vi "Sonicator Settings Dialog.vi"(8 "error in (no error)":errorcluster, 10 "Message Queues":T1, 11 "Sonicator Module State Cluster":T5={"State"=enum."Idle", "Start Time"=timestamp(0 s since 1904-01-01), "Current Time"=timestamp(0 s since 1904-01-01), "Sonicator Module Config"={"GUID"="", "Drop Coords"={"Horizontal"=0, "Vertical"=0}, "Process Name"="", "Queue Name"="", "Settings"={"Cycle Period"=500.0, "Sonicator Type"="Sonic Systems P100", "SS P100 Settings"={"VISA resource name"="", "Simulated?"=FALSE}, "Setpoint (µm)"=0.0, "Cutoff (µm)"=0.0}, "Load Count"=0}, "Output Error"=FALSE, "Log Started"=FALSE, "First Iteration"=FALSE, "Data"={"Sonicator Amp Value"=0.0, "Sonicator Power Value"=0.0}, "Sonicator On?"=enum."Off"}) -> (0 "error out":errorcluster, 1 "Cancelled?":bool=TRUE, 2 "UI Refresh Needed?":bool, 3 "Sonicator Module State Cluster":T5={"State"=enum."Idle", "Start Time"=timestamp(0 s since 1904-01-01), "Current Time"=timestamp(0 s since 1904-01-01), "Sonicator Module Config"={"GUID"="", "Drop Coords"={"Horizontal"=0, "Vertical"=0}, "Process Name"="", "Queue Name"="", "Settings"={"Cycle Period"=500.0, "Sonicator Type"="Sonic Systems P100", "SS P100 Settings"={"VISA resource name"="", "Simulated?"=FALSE}, "Setpoint (µm)"=0.0, "Cutoff (µm)"=0.0}, "Load Count"=0}, "Output Error"=FALSE, "Log Started"=FALSE, "First Iteration"=FALSE, "Data"={"Sonicator Amp Value"=0.0, "Sonicator Power Value"=0.0}, "Sonicator On?"=enum."Off"})   [LabVIEW 2018, in "Sonicator Module.lvlib"]
doc: "Dialog for selecting user specified settings."
uses:
  Sonicator Module.lvlib
  Feed Module/Controls/Sonicator Module State Cluster.ctl
  Pump Module Folder/Measure Instrument/State Enum.ctl
  Feed Module/Controls/Sonicator Module Config Cluster.ctl
  <vilib>/Utility/miscctls.llb/LVPoint32TypeDef.ctl
  Feed Module/Controls/Sonicator Module Settings Cluster.ctl
  Sonic Systems P100/Sonic Systems P100 Settings.ctl
  Feed Module/Controls/Sonicator Module Settings Cluster and Start Stop.ctl
  Sonicator Message Queues.ctl
  support/Message Queue/Message Cluster.ctl
  support/Message Queue/Enqueue Message (Single).vi
  <vilib>/Utility/xml.llb/Write to XML File(string).vi
  Settings/Settings.lvlib
  Measure Instrument/Sonicator Module Engine.lvlib
  support/Support Library.lvlib
  support/Message Queue/Message Queue.lvlib
  Sonic Systems P100/Sonic Systems P100.lvlib
  Pump Module Folder/Measure Instrument/Pump Module Engine.lvlib
panel:
  in  "Configuration + Buttons":T2={"Configuration"={"Cycle Period"=500.0, "Sonicator Type"="", "SS P100 Settings"={"VISA resource name"="", "Simulated?"=FALSE}, "Setpoint (µm)"=0.0, "Cutoff (µm)"=0.0}, "Stop"=FALSE, "Start"=FALSE}
  in  "Module Name":string
  in  "Cancel Button":bool
  in  "OK Button":bool
  # "Non visible portion of dialog (needed for connector pane)."
  # "Sonicator Settings"
  # "Sonicator Settings"
  # "Sonicator Settings"
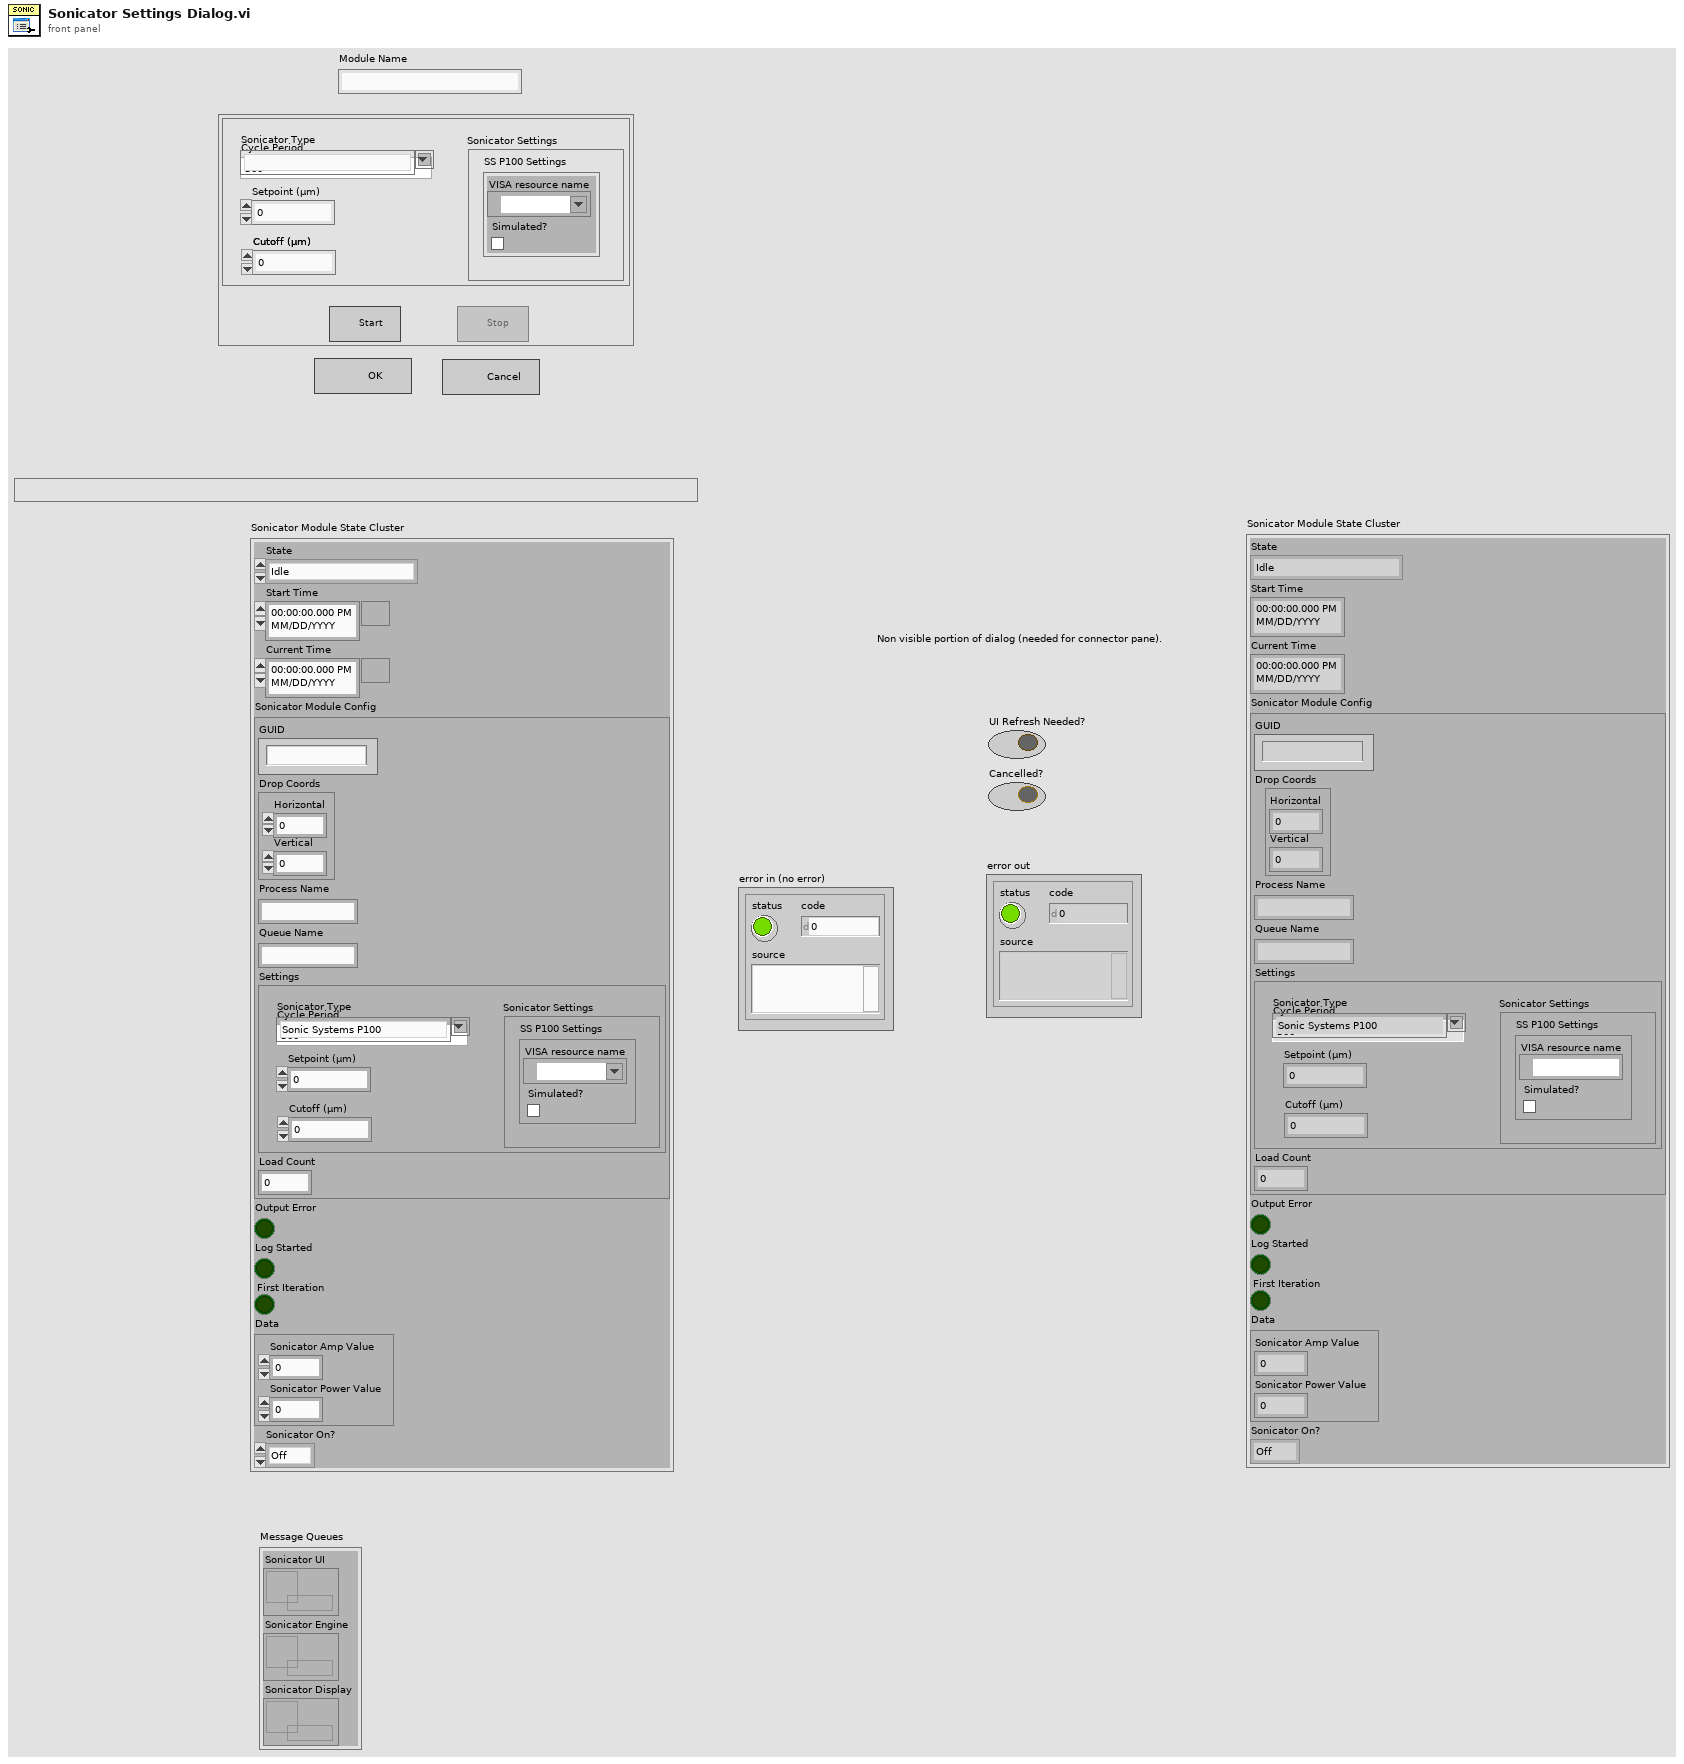
[diagram p1: front panel]
types:
  T1 = typedef "Sonicator Module.lvlib/Sonicator Message Queues.ctl" = cluster{"Sonicator UI":refnum<queue>, "Sonicator Engine":refnum<queue>, "Sonicator Display":refnum<queue>}
  T2 = typedef "Sonicator Module.lvlib/Sonicator Module Settings Cluster and Start Stop.ctl" = cluster{"Configuration":T3, "Stop":bool, "Start":bool}
  T3 = typedef "Sonicator Module.lvlib/Sonicator Module Settings Cluster.ctl" = cluster{"Cycle Period":dbl, "Sonicator Type":string, "SS P100 Settings":T4, "Setpoint (µm)":dbl, "Cutoff (µm)":dbl}
  T4 = typedef "Sonic Systems P100.lvlib/Sonic Systems P100 Settings.ctl" = cluster{"VISA resource name":refnum<visa-resource-name>, "Simulated?":bool}
  T5 = typedef "Sonicator Module.lvlib/Sonicator Module State Cluster.ctl" = cluster{"State":T6, "Start Time":timestamp, "Current Time":timestamp, "Sonicator Module Config":T7, "Output Error":bool, "Log Started":bool, "First Iteration":bool, "Data":cluster{"Sonicator Amp Value":dbl, "Sonicator Power Value":dbl}, "Sonicator On?":enum16{"Off", "On", "Not Initialized", "Over Cutoff"}}
  T6 = typedef "Pump Module.lvlib/Pump Module Engine.lvlib/State Enum.ctl" = enum16{"Measuring", "Idle", "Paused"}
  T7 = typedef "Sonicator Module.lvlib/Sonicator Module Config Cluster.ctl" = cluster{"GUID":string, "Drop Coords":T8, "Process Name":string, "Queue Name":string, "Settings":T3, "Load Count":i32}
  T8 = typedef "LVPoint32TypeDef.ctl" = cluster{"Horizontal":i32, "Vertical":i32}
  T9 = enum8{"Enabled", "Disabled", "Disabled and Grayed Out"}
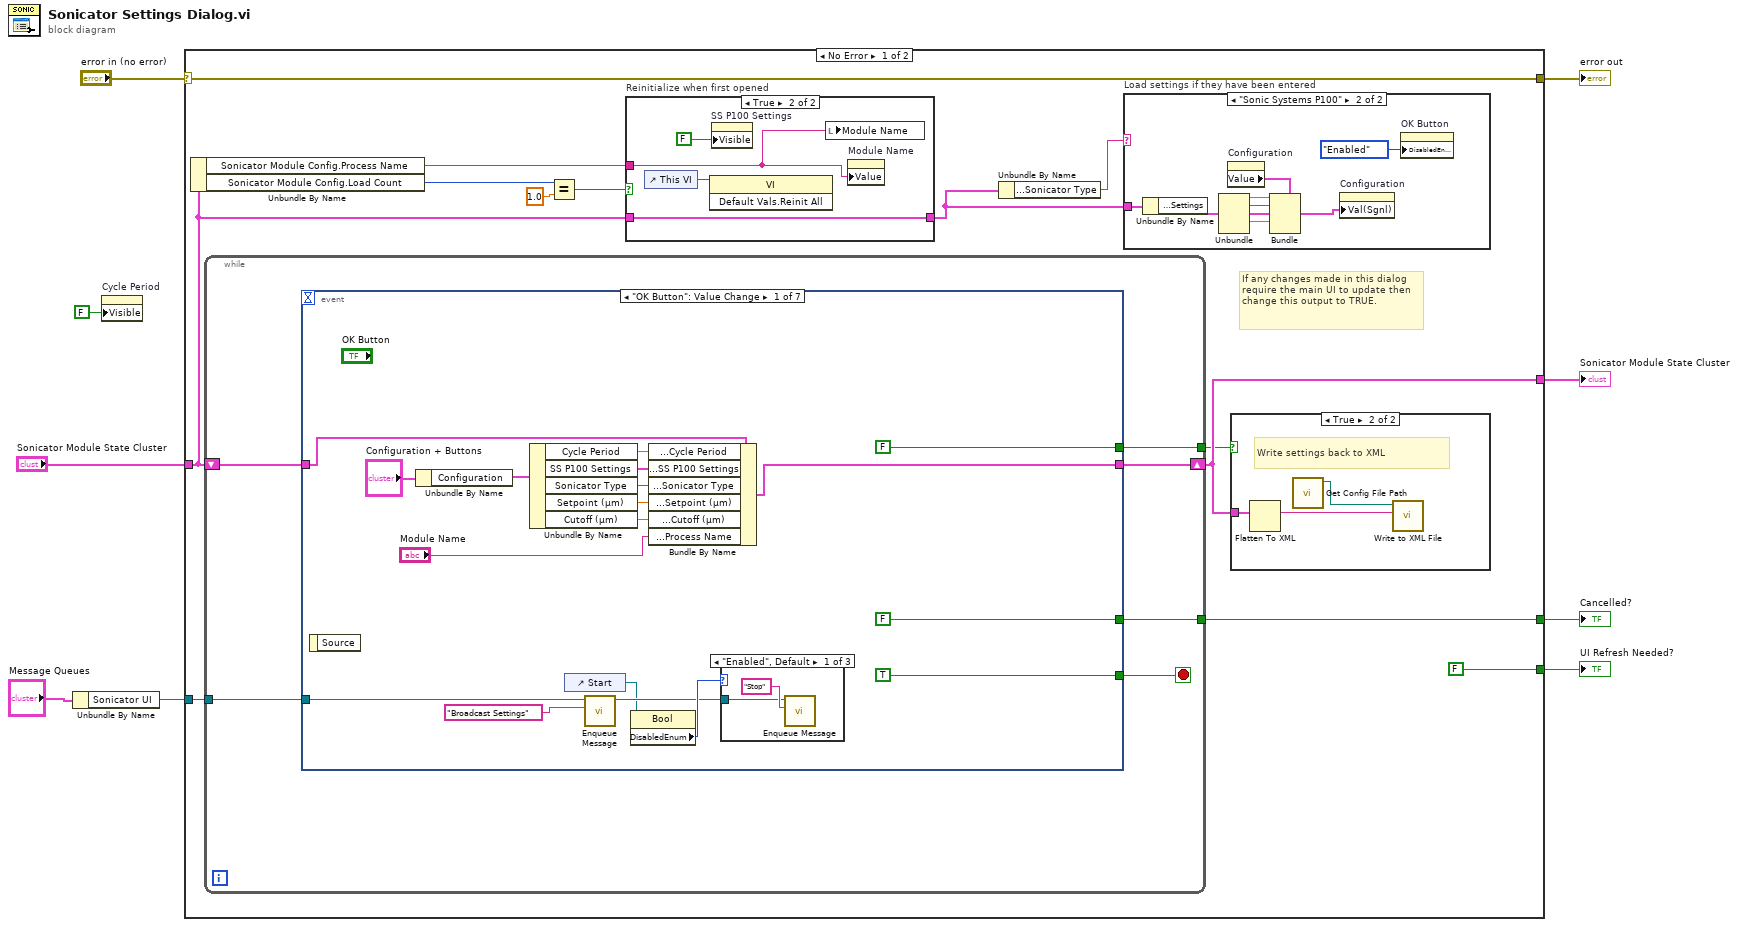
[diagram p0: block diagram]
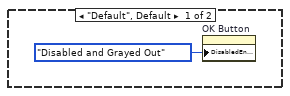
[diagram p2: hidden frame]
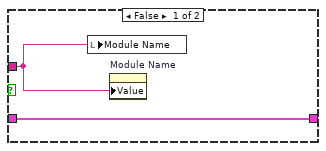
[diagram p3: hidden frame]
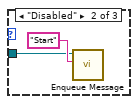
[diagram p4: hidden frame]
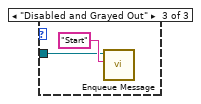
[diagram p5: hidden frame]
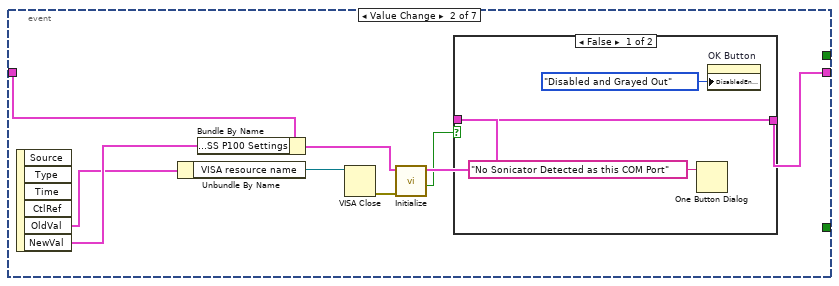
[diagram p6: hidden frame]
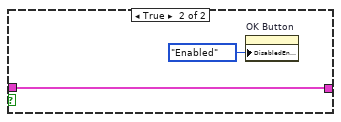
[diagram p7: hidden frame]
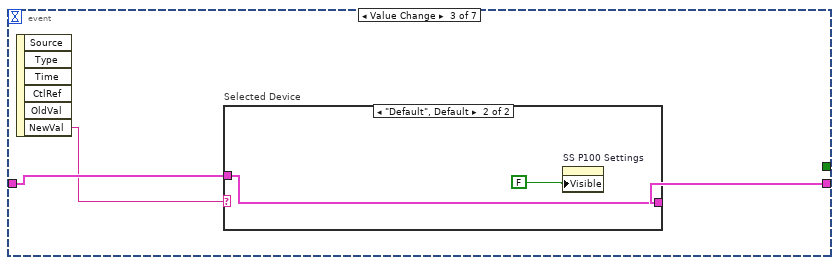
[diagram p8: hidden frame]
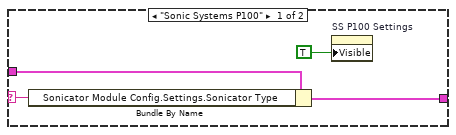
[diagram p9: hidden frame]
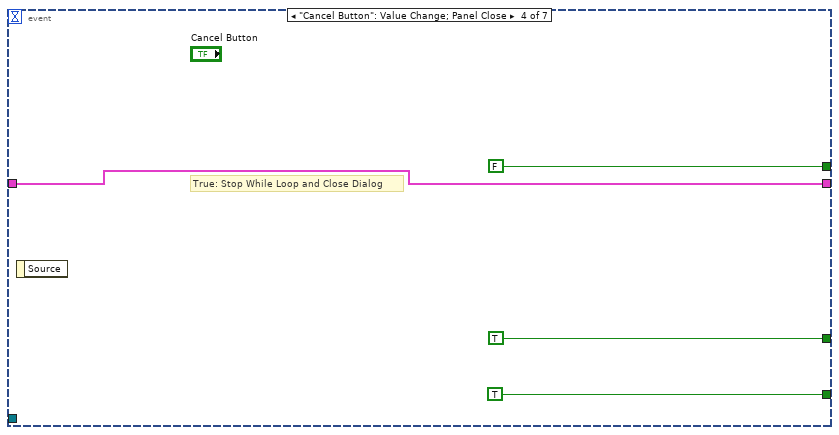
[diagram p10: hidden frame]
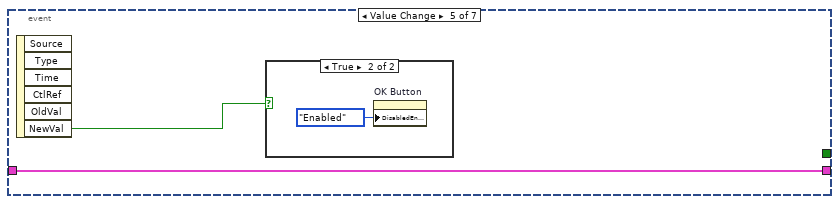
[diagram p11: hidden frame]
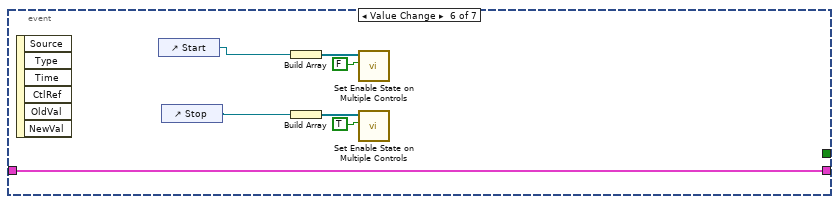
[diagram p13: hidden frame]
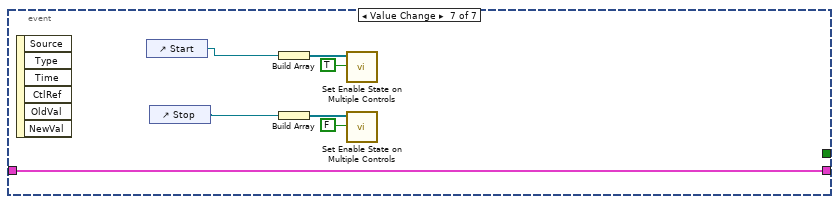
[diagram p14: hidden frame]
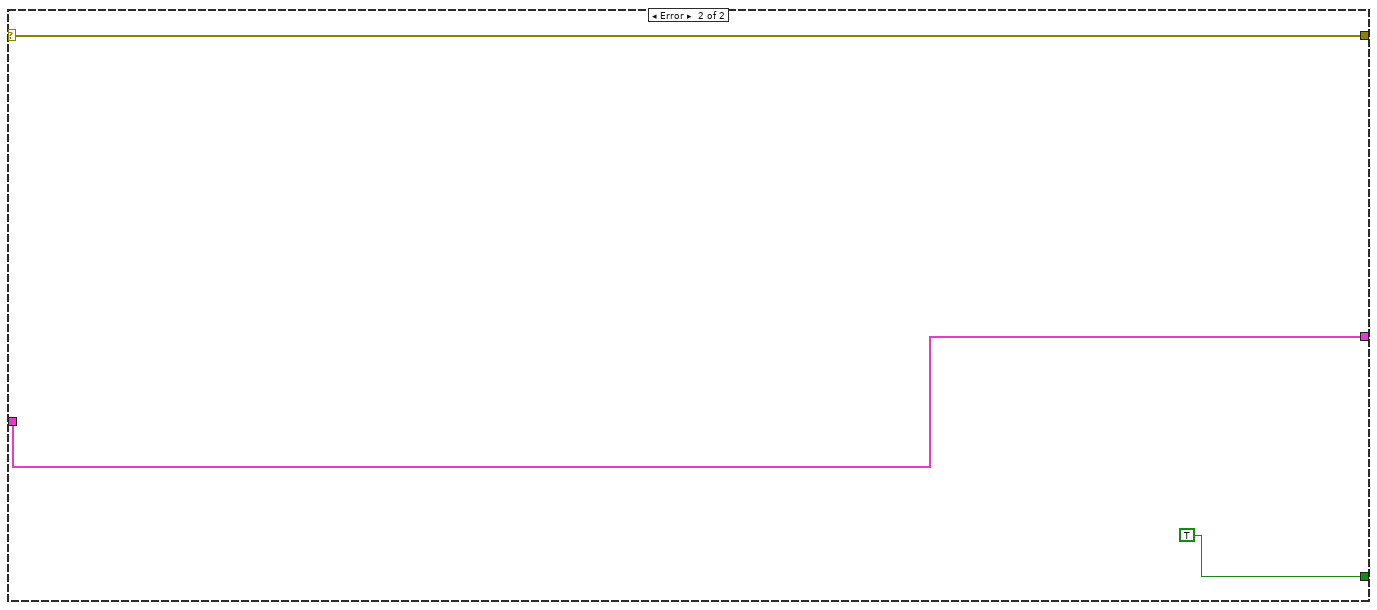
[diagram p16: hidden frame]
diagram:
  n1 = Unbundle By Name("Message Queues") -> ("Sonicator UI"=w1:refnum<queue>)
  n2 = property on="Cycle Period" class="DigNum (strict)"("Visible"=FALSE) -> ()  [unwired: 2 in, 2 out]
  n3 = case shown="No Error" "error in (no error)" {
    selector: "error in (no error)" -> [w22 w118]
    tunnel: [w22 w118] -> w9
    tunnel: "Sonicator Module State Cluster" -> [w12 w117]
    tunnel: [w20 w117] -> w4
    tunnel: [FALSE ("UI Refresh Needed?") _] -> w8
    tunnel: [w16 TRUE ("UI Refresh Needed?")] -> w7
    tunnel: w1 -> [w10 _]
    frame No Error {
      # "If any changes made in this dialog require the main UI to update then change this output to TRUE."
      n4 = Unbundle By Name(w12) -> ("Sonicator Module Config.Process Name"=w11:string, "Sonicator Module Config.Load Count"=w19:i32)
      n5 = while {
        tunnel: [w44] -> w17
        tunnel: [w41] -> w16
        shift-right: [w43] -> w20
        shift-left: w12 -> [w40]
        tunnel: w10 -> [w39]
        stop <- w42 stop-if-true
        n6 = event shown="[0] \"OK Button\": Value Change" {
          selector: _ -> [_ _ _ _ _ _ _]
          dyn-events: _ -> [_ _ _ _ _ _ _]
          timeout: _ -> [_ _ _ _ _ _ _]
          tunnel: [w60 w77 w83 w95 w97 w105 w112] -> w43
          tunnel: w40 -> [w57 w75 w85 w95 w97 w105 w112]
          tunnel: [FALSE ("UI Refresh Needed?") _ _ FALSE ("UI Refresh Needed?") _ _ _] -> w44
          tunnel: [TRUE _ _ TRUE _ _ _] -> w42
          tunnel: [FALSE ("UI Refresh Needed?") _ _ TRUE ("UI Refresh Needed?") _ _ _] -> w41
          tunnel: w39 -> [w47 _ _ _ _ _ _]
          event "OK Button": Value Change {
            n7 = event-data() -> ()  [unwired: 1 in, 1 out]
            n8 = Unbundle By Name("Configuration + Buttons") -> ("Configuration"=w53:T3)
            n9 = Unbundle By Name(w53) -> ("Cycle Period"=w58:dbl, "SS P100 Settings"=w56:T4, "Sonicator Type"=w55:string, "Setpoint (µm)"=w52:dbl, "Cutoff (µm)"=w45:dbl)
            n10 = control-ref of="Start"() -> (w48:refnum<vi>)
            n11 = call-poly "Enqueue Message.vi"("Message"="Broadcast Settings", "Message Queue"=w47) -> ("dup Message Queue"=w49:refnum<queue>)  [unwired: 8 in, 1 out]
            n12 = property class="Bool"(reference=w48) -> ("DisabledEnum"=w51:T9)  [unwired: 1 in, 2 out]
            n13 = Bundle By Name(cluster=w57, "Sonicator Module Config.Settings.Cycle Period"=w58, "Sonicator Module Config.Settings.SS P100 Settings"=w56, "Sonicator Module Config.Settings.Sonicator Type"=w55, "Sonicator Module Config.Settings.Setpoint (µm)"=w52, "Sonicator Module Config.Settings.Cutoff (µm)"=w45, "Sonicator Module Config.Process Name"="Module Name") -> (w60:T5)
            n14 = case shown="\"Enabled\", Default" w51 {
              tunnel: w49 -> [w63 w65 w67]
              frame "Enabled", Default {
                n15 = call-poly "Enqueue Message.vi"("Message"="Stop", "Message Queue"=w63) -> ()  [unwired: 8 in, 2 out]
              }
              frame "Disabled" {
                n16 = call-poly "Enqueue Message.vi"("Message"="Start", "Message Queue"=w65) -> ()  [unwired: 8 in, 2 out]
              }
              frame "Disabled and Grayed Out" {
                n17 = call-poly "Enqueue Message.vi"("Message"="Start", "Message Queue"=w67) -> ()  [unwired: 8 in, 2 out]
              }
            }
          }
          event Value Change {
            n18 = event-data() -> ("OldVal"=w69:T4, "NewVal"=w71:T4)  [unwired: 1 in, 4 out]
            n19 = Unbundle By Name(w69) -> ("VISA resource name"=w70:refnum<visa-resource-name>)
            n20 = Bundle By Name(cluster=w75, "Sonicator Module Config.Settings.SS P100 Settings"=w71) -> (w74:T5)
            n21 = VISA Close(VISA resource name=w70) -> (error out=w76:errorcluster)  [unwired: 1 in]
            n22 = call "Initialize.vi"("error in (no error)"=w76, "Sonicator Module State Cluster"=w74) -> ("Initialized"=w72:bool, "Sonicator Module State Cluster"=w73:T5)  [unwired: 7 in, 1 out]
            n23 = case shown="False" w72 {
              tunnel: [w79 w81] -> w77
              tunnel: w73 -> [w79 w81]
              frame False {
                n24 = One Button Dialog(message="No Sonicator Detected as this COM Port") -> ()  [unwired: 1 in, 1 out]
                n25 = property on="OK Button" class="Bool"("DisabledEnum"=T9."Disabled and Grayed Out" ("Disabled")) -> ()  [unwired: 2 in, 2 out]
              }
              frame True {
                n26 = property on="OK Button" class="Bool"("DisabledEnum"=T9."Enabled" ("Disabled")) -> ()  [unwired: 2 in, 2 out]
              }
            }
          }
          event Value Change {
            n27 = event-data() -> ("NewVal"=w84:string)  [unwired: 1 in, 5 out]
            n28 = case "Selected Device" shown="\"Default\", Default" w84 {
              selector: w84 -> [w87 _]
              tunnel: w85 -> [w89 w91]
              tunnel: [w88 w91] -> w83
              frame "Sonic Systems P100" {
                n29 = Bundle By Name(cluster=w89, "Sonicator Module Config.Settings.Sonicator Type"=w87) -> (w88:T5)
                n30 = property on="SS P100 Settings" class="Clust (strict)"("Visible"=TRUE) -> ()  [unwired: 2 in, 2 out]
              }
              frame "Default", Default {
                n31 = property on="SS P100 Settings" class="Clust (strict)"("Visible"=FALSE) -> ()  [unwired: 2 in, 2 out]
              }
            }
          }
          event "Cancel Button": Value Change; Panel Close {
            # "True: Stop While Loop and Close Dialog"
            n32 = event-data() -> ()  [unwired: 1 in, 1 out]
          }
          event Value Change {
            n33 = event-data() -> ("NewVal"=w96:bool)  [unwired: 1 in, 5 out]
            n34 = case shown="True" w96 {
              frame False {
              }
              frame True {
                n35 = property on="OK Button" class="Bool"("DisabledEnum"=T9."Enabled" ("Disabled")) -> ()  [unwired: 2 in, 2 out]
              }
            }
          }
          event Value Change {
            n36 = event-data() -> ()  [unwired: 1 in, 6 out]
            n37 = control-ref of="Start"() -> (w100:refnum<vi>)
            n38 = control-ref of="Stop"() -> (w99:refnum<vi>)
            n39 = Build Array(w100) -> (w102:refnum<vi>[])
            n40 = Build Array(w99) -> (w104:refnum<vi>[])
            n41 = call "Set Enable State on Multiple Controls.vi"("Enable?"=FALSE, "Controls"=w102) -> ()  [unwired: 10 in]
            n42 = call "Set Enable State on Multiple Controls.vi"("Enable?"=TRUE, "Controls"=w104) -> ()  [unwired: 10 in]
          }
          event Value Change {
            n43 = event-data() -> ()  [unwired: 1 in, 6 out]
            n44 = control-ref of="Start"() -> (w109:refnum<vi>)
            n45 = control-ref of="Stop"() -> (w108:refnum<vi>)
            n46 = Build Array(w109) -> (w110:refnum<vi>[])
            n47 = Build Array(w108) -> (w111:refnum<vi>[])
            n48 = call "Set Enable State on Multiple Controls.vi"("Enable?"=TRUE, "Controls"=w110) -> ()  [unwired: 10 in]
            n49 = call "Set Enable State on Multiple Controls.vi"("Enable?"=FALSE, "Controls"=w111) -> ()  [unwired: 10 in]
          }
        }
      }
      n50 = Equal?(x=w19, y=1.0) -> (x = y?=w15:bool)
      n51 = case "Reinitialize when first opened" shown="True" w15 {
        tunnel: w12 -> [w34 w37]
        tunnel: [w34 w37] -> w13
        tunnel: w11 -> [w33 w36]
        frame False {
          n52 = local write "Module Name"(w33) -> ()
          n53 = property on="Module Name" class="Str"("Value"=w33) -> ()  [unwired: 2 in, 2 out]
        }
        frame True {
          n54 = control-ref of="This VI"() -> (w38:refnum<vi>)
          n55 = invoke class="VI" method="Default Vals.Reinit All"(reference=w38) -> ()  [unwired: 2 in, 3 out]
          n56 = property on="SS P100 Settings" class="Clust (strict)"("Visible"=FALSE) -> ()  [unwired: 2 in, 2 out]
          n57 = local write "Module Name"(w36) -> ()
          n58 = property on="Module Name" class="Str"("Value"=w36) -> ()  [unwired: 2 in, 2 out]
        }
      }
      n59 = Unbundle By Name(w13) -> ("Sonicator Module Config.Settings.Sonicator Type"=w14:string)
      n60 = case "Load settings if they have been entered" shown="\"Sonic Systems P100\"" w14 {
        tunnel: w13 -> [_ w28]
        frame "Default", Default {
          n61 = property on="OK Button" class="Bool"("DisabledEnum"=T9."Disabled and Grayed Out" ("Disabled")) -> ()  [unwired: 2 in, 2 out]
        }
        frame "Sonic Systems P100" {
          n62 = Unbundle By Name(w28) -> ("Sonicator Module Config.Settings"=w30:T3)
          n63 = Unbundle(w30) -> ("Cycle Period"=w31:dbl, "Sonicator Type"=w32:string, "SS P100 Settings"=w29:T4, "Setpoint (µm)"=w26:dbl)  [unwired: 1 out]
          n64 = property on="Configuration" class="Clust (strict)"() -> ("Value"=w25:T3)  [unwired: 2 in, 2 out]
          n65 = Bundle(cluster=w25, "Cycle Period"=w31, "Sonicator Type"=w32, "SS P100 Settings"=w29, "Setpoint (µm)"=w26) -> (w24:T3)  [unwired: 1 in]
          n66 = property on="Configuration" class="Clust (strict)"("Val(Sgnl)"=w24) -> ()  [unwired: 2 in, 2 out]
          n67 = property on="OK Button" class="Bool"("DisabledEnum"=T9."Enabled" ("Disabled")) -> ()  [unwired: 2 in, 2 out]
        }
      }
      n68 = case shown="True" w17 {
        tunnel: w20 -> [_ w114]
        frame False {
        }
        frame True {
          # "Write settings back to XML"
          n69 = Flatten To XML(anything=w114) -> (xml string=w113:string)
          n70 = call "Get Config File Path.vi"() -> ("XML File Path"=w115:path)  [unwired: 10 in, 1 out]
          n71 = call-poly <vilib>:"Write to XML File.vi"("XML Input"=w113, "XML File Path"=w115) -> ()  [unwired: 7 in, 3 out]
        }
      }
    }
    frame Error {
    }
  }
  "UI Refresh Needed?" <- w8
  "error out" <- w9
  "Cancelled?" <- w7
  "Sonicator Module State Cluster" <- w4
